vi "WriteMeasData.vi"(8 "error in (no error)":errorcluster, 10 "Data Cluster":T1, 11 "Byte Stream File in":refnum<file>) -> (0 "error out":errorcluster, 3 "Byte Stream File out":refnum<file>)   [LabVIEW 2017]
uses:
  Controls/DataCluster.ctl
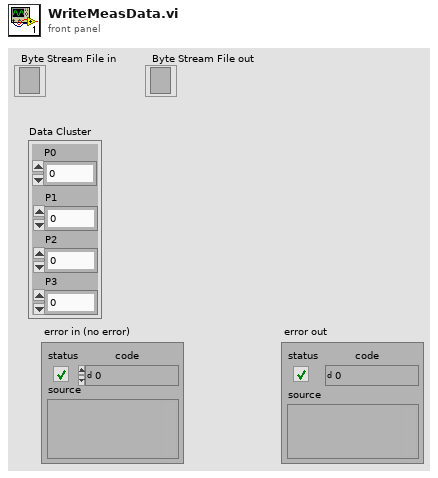
[diagram p1: front panel]
types:
  T1 = typedef "DataCluster.ctl" = cluster{"P0":dbl, "P1":dbl, "P2":dbl, "P3":dbl}
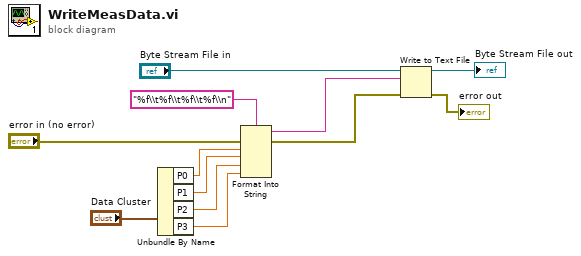
[diagram p0: block diagram]
diagram:
  n1 = Unbundle By Name("Data Cluster") -> ("P0"=w4:dbl, "P1"=w3:dbl, "P2"=w2:dbl, "P3"=w1:dbl)
  n2 = Format Into String(format string="%f\\t%f\\t%f\\t%f\\n", error in="error in (no error)", w4, w3, w2, w1) -> (resulting string=w8:string, error out=w6:errorcluster)  [unwired: 1 in]
  n3 = Write to Text File(file (use dialog)="Byte Stream File in", text=w8, error in=w6) -> (refnum out=→"Byte Stream File out":refnum<file>, error out=→"error out":errorcluster)  [unwired: 1 in, 1 out]
